vi "ToString.vi"(0 "reference in":refnum<class "MyDemoClass.lvclass">, 5 "error in (no error)":errorcluster) -> (14 "reference out":refnum<class "MyDemoClass.lvclass">, 15 "string":string, 19 "error out":errorcluster)   [LabVIEW 2017, in "MyDemoClass.lvclass"]
uses:
  MyDemoClass.lvclass
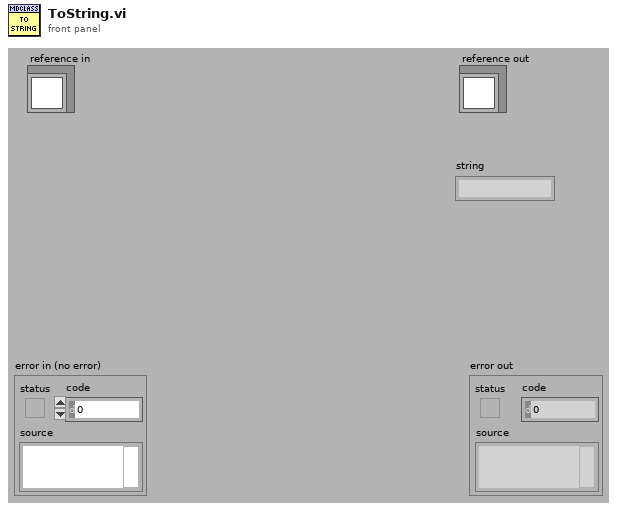
[diagram p1: front panel]
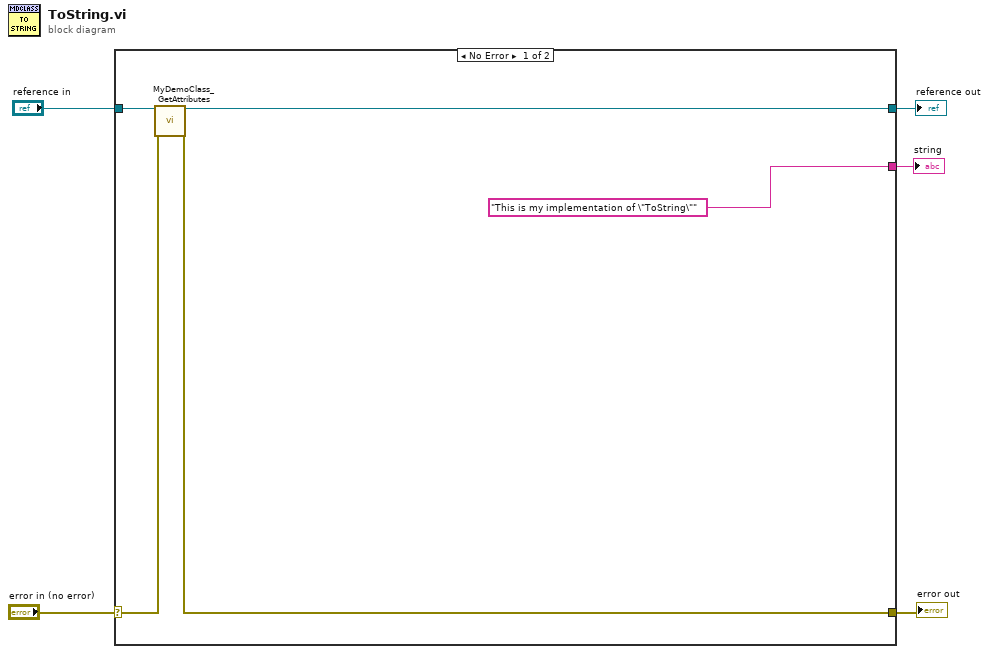
[diagram p0: block diagram]
diagram:
  n1 = case shown="No Error" "error in (no error)" {
    selector: "error in (no error)" -> [w10 w12]
    tunnel: [w9 w12] -> w4
    tunnel: [w7 w11] -> w2
    tunnel: "reference in" -> [w8 w11]
    tunnel: ["This is my implementation of \"ToString\"" _] -> w1
    frame No Error {
      n2 = call "MyDemoClass_GetAttributes.vi"("reference in"=w8, "error in (no error)"=w10) -> ("reference out"=w7:refnum<class "MyDemoClass.lvclass">, "error out"=w9:errorcluster)  [unwired: 14 in, 2 out]
    }
    frame Error {
    }
  }
  "error out" <- w4
  "reference out" <- w2
  "string" <- w1
